vi "Construct Field Child by Ctrl Class.vi"(8 "error in (no error)":errorcluster, 11 "Field in":refnum<class "Field.lvclass">) -> (0 "error out":errorcluster, 3 "Field out":refnum<class "Field.lvclass">)   [LabVIEW 2020, in "Field.lvclass"]
uses:
  Field.lvclass
  Numeric Field/Numeric Field.lvclass
  C:/Users/User/Desktop/Raman Program/Database OOP/source/Field/Field.lvclass
  Test field/Text field.lvclass
  Ring Field/Ring Field.lvclass
  Field.lvclass/Field.ctl
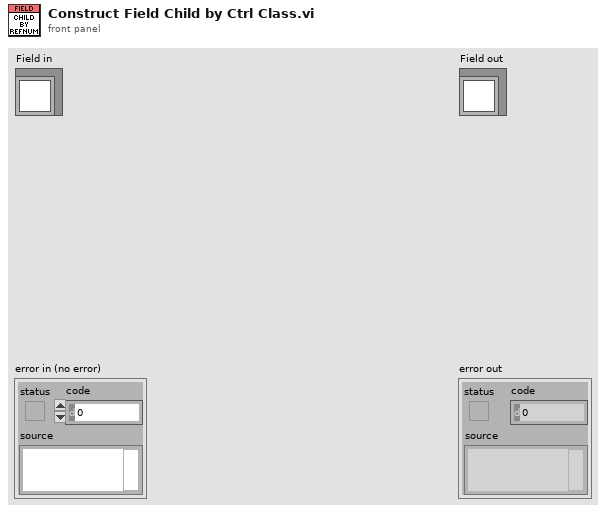
[diagram p1: front panel]
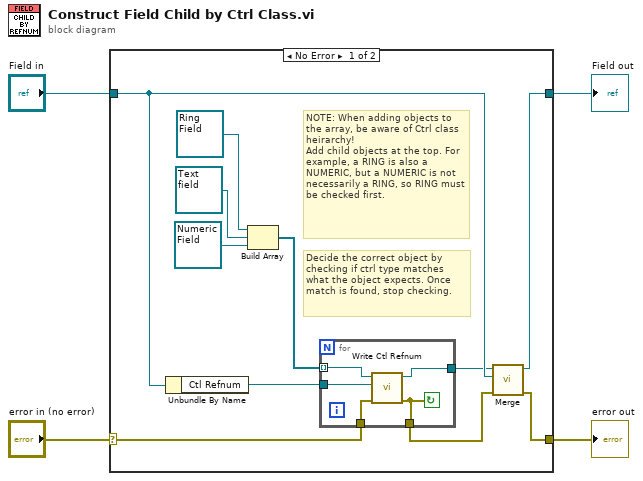
[diagram p0: block diagram]
diagram:
  n1 = case shown="No Error" "error in (no error)" {
    selector: "error in (no error)" -> [w7 w22]
    tunnel: [w5 w22] -> w3
    tunnel: [w8 w21] -> w1
    tunnel: "Field in" -> [w10 w21]
    frame No Error {
      # "Decide the correct object by\nchecking if ctrl type matches\nwhat the object expects. Once match is found, stop checking."
      # "NOTE: When adding objects to the array, be aware of Ctrl class heirarchy!\nAdd child objects at the top. For example, a RING is also a NUMERIC, but a NUMERIC is not necessarily a RING, so RING must be checked first."
      n2 = Unbundle By Name(w10) -> ("Ctl Refnum"=w15:refnum<vi>)
      n3 = Build Array(refnum<class "Ring Field.lvclass"> refnum ("Ring Field.lvclass"), refnum<class "Text field.lvclass"> refnum ("Text field.lvclass"), refnum<class "Numeric Field.lvclass"> refnum ("Numeric Field.lvclass")) -> (w11:refnum<class "Field.lvclass">[])
      n4 = for {
        tunnel: w15 -> [w20]
        tunnel: [w19] -> w9
        tunnel: w11 -> [w18] mode=indexing
        tunnel: w7 -> [w17]
        tunnel: [w16] -> w6
        stop <- w16 continue-if-true
        n5 = call "Write Ctl Refnum.vi"("error in (no error)"=w17, "Ctl Refnum"=w20, "Field in"=w18) -> ("error out"=w16:errorcluster, "Field out"=w19:refnum<class "Field.lvclass">)  [unwired: 7 in]
      }
      n6 = call-dynamic "Merge.vi"("error in (no error)"=w6, "Field To Merge"=w10, "Field In"=w9) -> ("error out"=w5:errorcluster, "Merged Field out"=w8:refnum<class "Field.lvclass">)  [unwired: 7 in]
    }
    frame Error {
    }
  }
  "error out" <- w3
  "Field out" <- w1
